vi "Assert Log File Size.vi"(8 "error in (no error)":errorcluster, 11 "Embedded Data Logger System Tests in":refnum<class "Embedded Data Logger System Tests.lvclass">) -> (0 "error out":errorcluster, 3 "Embedded Data Logger System Tests out":refnum<class "Embedded Data Logger System Tests.lvclass">)   [LabVIEW 2018, in "Embedded Data Logger System Tests.lvclass"]
uses:
  Embedded Data Logger System Tests.lvclass
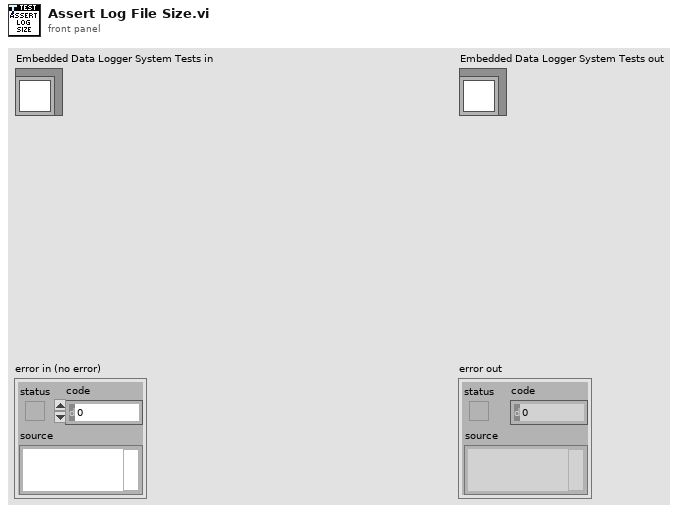
[diagram p1: front panel]
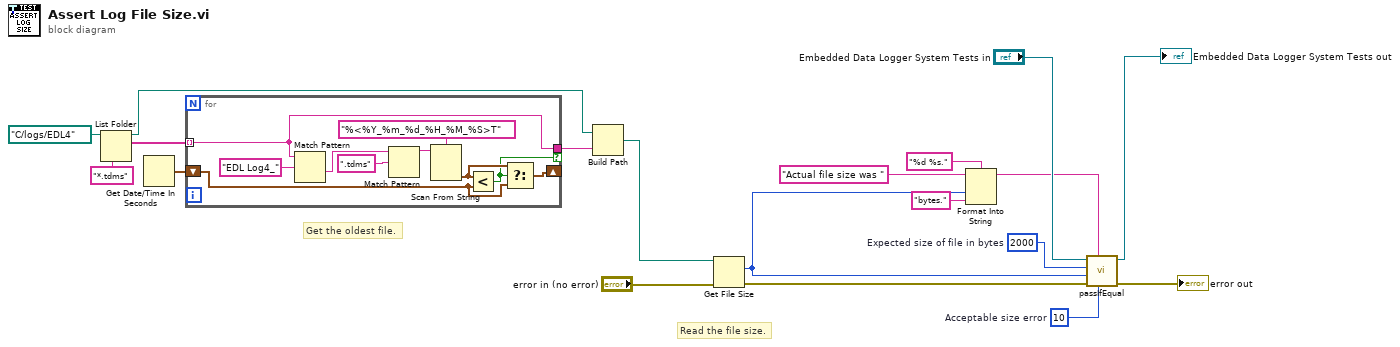
[diagram p0: block diagram]
diagram:
  w5 = i64 10  # Acceptable size error
  w6 = i64 2000  # Expected size of file in bytes
  # "Read the file size."
  # "Get the oldest file."
  n1 = List Folder(path=path "C:/logs/EDL4" ("file path"), pattern="*.tdms") -> (path out=w16:path, filenames=w19:string[])  [unwired: 2 in, 2 out]
  n2 = Get Date/Time In Seconds() -> (seconds since 1Jan1904=w18:timestamp)
  n3 = for {
    tunnel: w19 -> [w24] mode=indexing
    shift-right: [w25] -> _
    shift-left: w18 -> [w26]
    tunnel: [w24] -> w17 if=w23
    n4 = Match Pattern(string=w24, regular expression="EDL Log4_") -> (after substring=w22:string)  [unwired: 1 in, 3 out]
    n5 = Match Pattern(string=w22, regular expression=".tdms") -> (before substring=w20:string)  [unwired: 1 in, 3 out]
    n6 = Scan From String(format string="%<%Y_%m_%d_%H_%M_%S>T", input string=w20) -> (output 1=w27:timestamp)  [unwired: 3 in, 3 out]
    n7 = Less?(x=w27, y=w26) -> (x < y?=w23:bool)
    n8 = Select(t=w27, s=w23, f=w26) -> (s? t:f=w25:timestamp)
  }
  n9 = Build Path(base path=w16, name or relative path=w17) -> (appended path=w7:path)
  n10 = Get File Size(file=w7, error in="error in (no error)") -> (size (in bytes)=w1:i64, 0:w2:errorcluster)  [unwired: 1 out]
  n11 = Format Into String(format string="%d %s.", initial string="Actual file size was ", w1, "bytes." ("input 2")) -> (resulting string=w8:string)  [unwired: 1 in, 1 out]
  n12 = call-dynamic "passIfEqual.vi"("delta (optional)"=w5, "custom report message (\"\")"=w8, "error in (no error)"=w2, "y"=w1, "x"=w6, "TestCase in"="Embedded Data Logger System Tests in") -> ("error out"=→"error out":errorcluster, "TestCase out"=→"Embedded Data Logger System Tests out":refnum<class "Embedded Data Logger System Tests.lvclass">)  [unwired: 4 in]
